vi "Read Ver.vi"(11 "SMSD ADU in":refnum<class "SMSD ADU.lvclass">) -> (2 "Ver":u8=1, 3 "SMSD ADU out":refnum<class "SMSD ADU.lvclass">)   [LabVIEW 2021, in "SMSD ADU.lvclass"]
uses:
  SMSD ADU.lvclass
  SMSD ADU.lvclass/SMSD ADU.ctl
panel:
  out "error out":errorcluster
  in  "error in (no error)":errorcluster
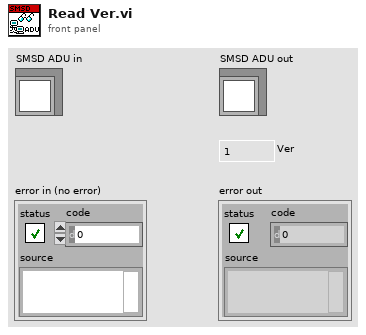
[diagram p1: front panel]
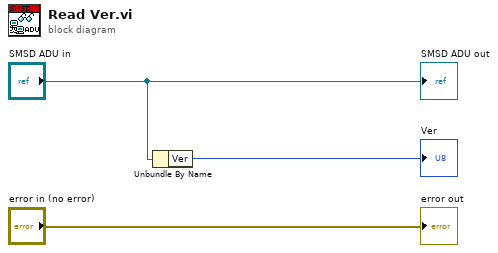
[diagram p0: block diagram]
diagram:
  n1 = Unbundle By Name("SMSD ADU in") -> ("Ver"=→"Ver":u8)
  "SMSD ADU out" <- "SMSD ADU in"
  "error out" <- "error in (no error)"
